vi "Init Options Dialog.vi"(6 "Controls":refnum<vi>[](array[refnum]), 11 "Options":T1) -> (3 "Init Steps":string[](array[string]))   [LabVIEW 2011]
uses:
  Controls/Options.ctl
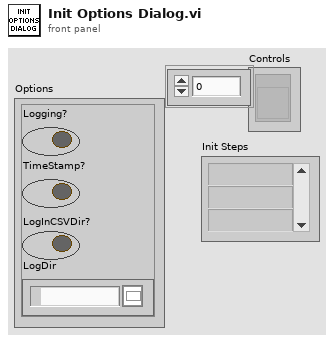
[diagram p1: front panel]
types:
  T1 = typedef "Options.ctl" = cluster{"Logging?":bool, "TimeStamp?":bool, "LogInCSVDir?":bool, "LogDir":path}
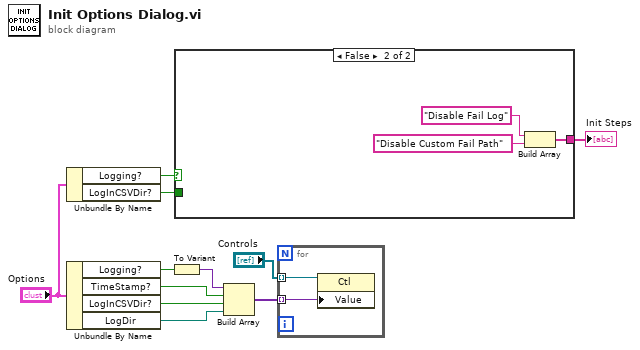
[diagram p0: block diagram]
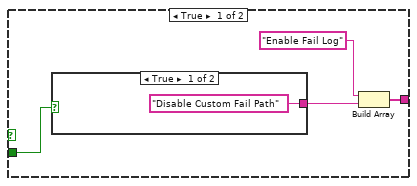
[diagram p2: hidden frame]
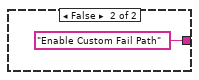
[diagram p3: hidden frame]
diagram:
  n1 = Unbundle By Name("Options") -> ("Logging?"=w11:bool, "LogInCSVDir?"=w2:bool)
  n2 = Unbundle By Name("Options") -> ("Logging?"=w8:bool, "TimeStamp?"=w6:bool, "LogInCSVDir?"=w5:bool, "LogDir"=w4:path)
  n3 = To Variant(anything=w8) -> (Variant=w7:variant)
  n4 = case shown="False" w11 {
    tunnel: [w12 w19] -> w1
    tunnel: w2 -> [w15 _]
    frame True {
      n5 = case shown="True" w15 {
        tunnel: ["Disable Custom Fail Path" "Enable Custom Fail Path"] -> w13
        frame True {
        }
        frame False {
        }
      }
      n6 = Build Array("Enable Fail Log", w13) -> (w12:string[])
    }
    frame False {
      n7 = Build Array("Disable Fail Log", "Disable Custom Fail Path") -> (w19:string[])
    }
  }
  "Init Steps" <- w1
  n8 = Build Array(w7, w6, w5, w4) -> (w3:variant[])
  n9 = for {
    tunnel: "Controls" -> [w22] mode=indexing
    tunnel: w3 -> [w21] mode=indexing
    n10 = property class="Ctl"(reference=w22, "Value"=w21) -> ()  [unwired: 1 in, 2 out]
  }
